vi "SRV_File Name and Extension (String).vi"(10 "File or Directory String":string) -> (1 "Extension":string, 2 "Name":string)   [LabVIEW 2009]
doc: "For a specified file or directory string, returns the file's or directory's name (i.e., the full input path with the file's or directory's extension stripped off) and extension.\n\nNote: this simply searches for the final period of the input string; it does not check for illegal characters or improperly-formed paths.\n\n\nAuthor: Mike Schultz - Logic PD"
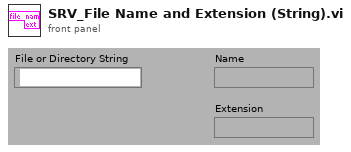
[diagram p1: front panel]
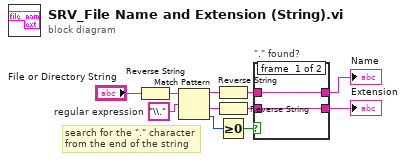
[diagram p0: block diagram]
diagram:
  w10 = "\\."  # regular expression
  # "search for the \".\" character from the end of the string"
  n1 = Reverse String(1:"File or Directory String") -> (0:w9:string)
  n2 = Match Pattern(string=w9, regular expression=w10) -> (before substring=w6:string, after substring=w5:string, offset past match=w8:i32)  [unwired: 2 out]
  n3 = Reverse String(1:w6) -> (0:w4:string)
  n4 = Reverse String(1:w5) -> (0:w3:string)
  n5 = Greater Or Equal To 0?(x=w8) -> (x >= 0?=w7:bool)
  n6 = case "\".\" found?" shown="False" w7 {
    tunnel: [w13 w14] -> w1
    tunnel: w4 -> [w13 w15]
    tunnel: [w12 w15] -> w11
    tunnel: w3 -> [w12 w14]
    frame #0 {
    }
    frame #1 {
    }
  }
  "Name" <- w1
  "Extension" <- w11
